vi "angleDifference.vi"(10 "theta B":dbl, 11 "theta A":dbl) -> (3 "delta theta":dbl)   [LabVIEW 2016]
uses:
  <vilib>/Analysis/coordinate.llb/Angle Units.ctl
  <vilib>/Analysis/coordinate.llb/Angle Range (Degree).ctl
  <vilib>/Analysis/coordinate.llb/Wrap Angle (scalar).vi
  <vilib>/Analysis/NI_AAL_Angle.lvlib
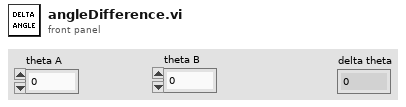
[diagram p1: front panel]
types:
  T1 = typedef "NI_AAL_Angle.lvlib/Angle Range (Degree).ctl" = u16
  T2 = typedef "NI_AAL_Angle.lvlib/Angle Units.ctl" = i32
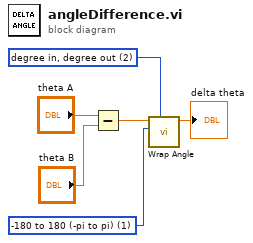
[diagram p0: block diagram]
diagram:
  w5 = T1 1 items=["none", "-180 to 180 (-pi to pi)", "0 to 360 (0 to 2pi)"] ("angle range")
  w6 = T2 2 items=["radian in, radian out", "radian in, degree out", "degree in, degree out", "degree in, radian out"] ("angle units")
  n1 = Subtract(x="theta A", y="theta B") -> (x-y=w2:dbl)
  n2 = call-poly <vilib>:"Wrap Angle.vi"("angle units"=w6, "angle range"=w5, "angle in"=w2) -> ("angle out"=→"delta theta":dbl)  [unwired: 7 in, 1 out]
